vi "Otm Acquisition Loop.vi"(8 "error in (no error)":errorcluster, 9 "Data Queue":refnum<queue>, 10 "Data Notifier":refnum<notifier>, 11 "Message Queues":T1) -> (0 "error out":errorcluster)   [LabVIEW 2017]
doc: "Message loop for handling messages pertaining to the acquisition of data from the hardware."
uses:
  support/Message Queue/All Message Queues.ctl
  support/Message Queue/Message Cluster.ctl
  Acquisition/Hardware Configuration.ctl
  Acquisition/Signal Type.ctl
  Acquisition/Acquisition State.ctl
  support/Message Queue/Enqueue Message (Single).vi
  <vilib>/Utility/error.llb/Error Cluster From Error Code.vi
  <vilib>/ErrorRing/Error Ring.xnode
  Acquisition/Acquisition.lvlib
  support/Message Queue/Message Queue.lvlib
panel:
  in  "扫描频率":dbl
  out "运行时间":dbl
  in  "测试时间":dbl=30.0
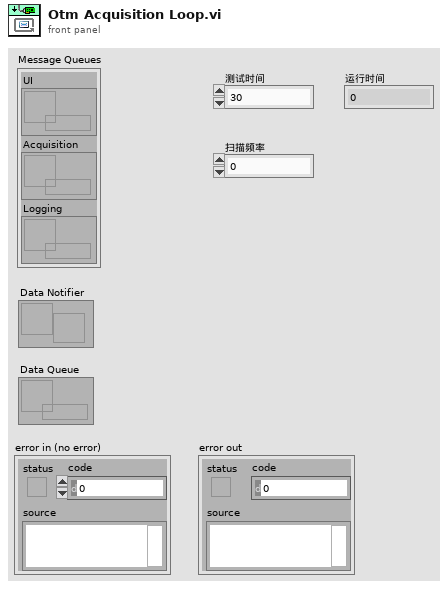
[diagram p1: front panel]
types:
  T1 = typedef "Message Queue.lvlib/All Message Queues.ctl" = cluster{"UI":refnum<queue>, "Acquisition":refnum<queue>, "Logging":refnum<queue>}
  T2 = typedef "Acquisition.lvlib/Hardware Configuration.ctl" = cluster{"HW Refnum <Replace Me>":string, "Signal Type <Replace Me>":T3}
  T3 = typedef "Acquisition.lvlib/Signal Type.ctl" = enum16{"Sine Wave", "Square with Noise"}
  T4 = typedef "Acquisition.lvlib/Acquisition State.ctl" = enum16{"Idle", "Acquiring"}
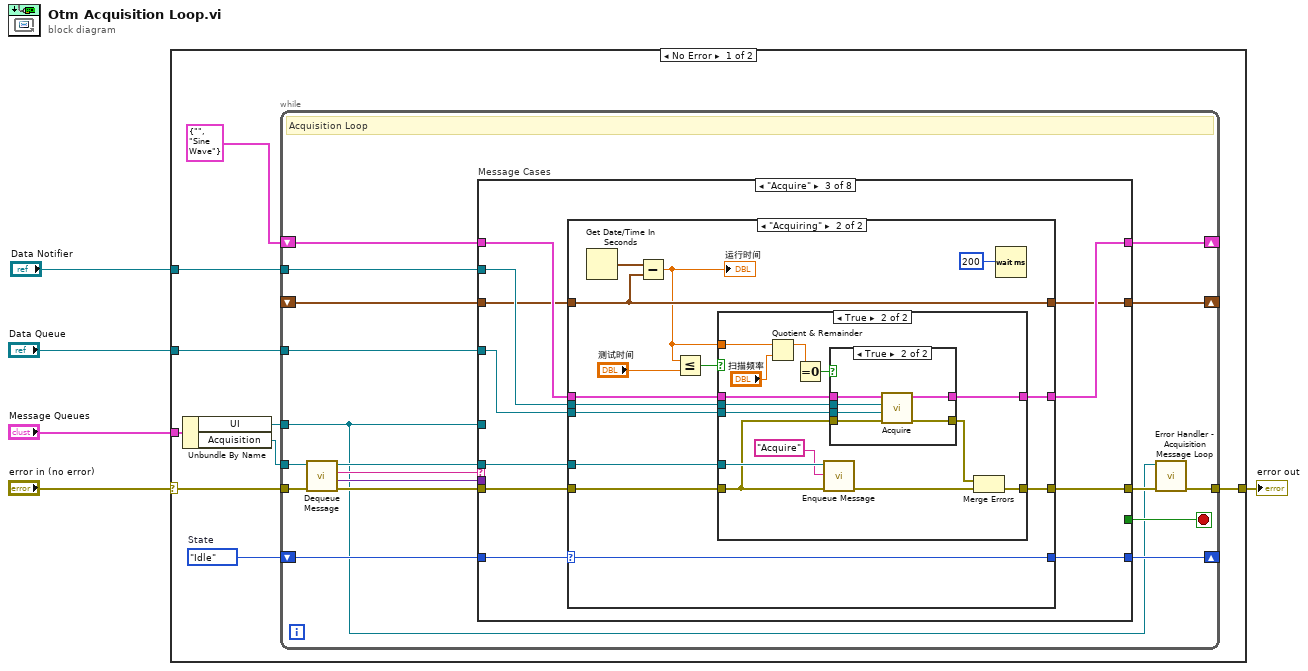
[diagram p0: block diagram]
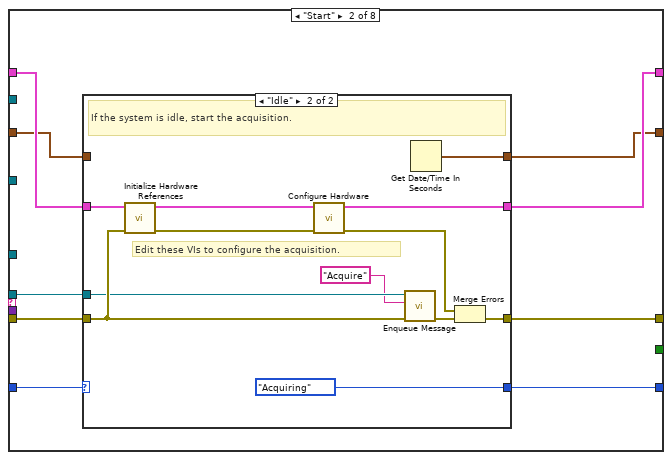
[diagram p3: hidden frame]
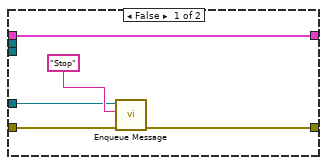
[diagram p6: hidden frame]
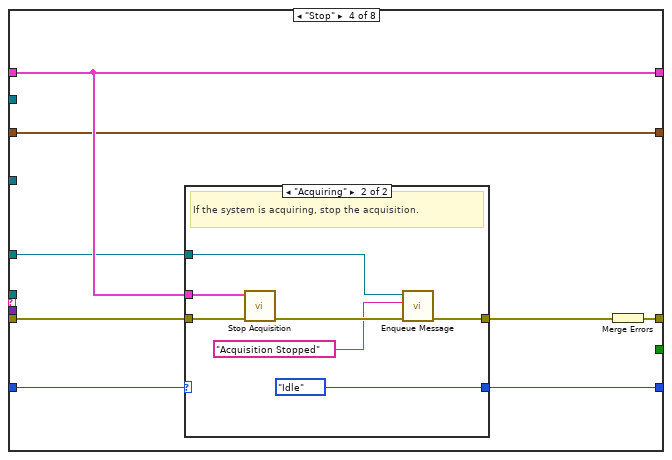
[diagram p8: hidden frame]
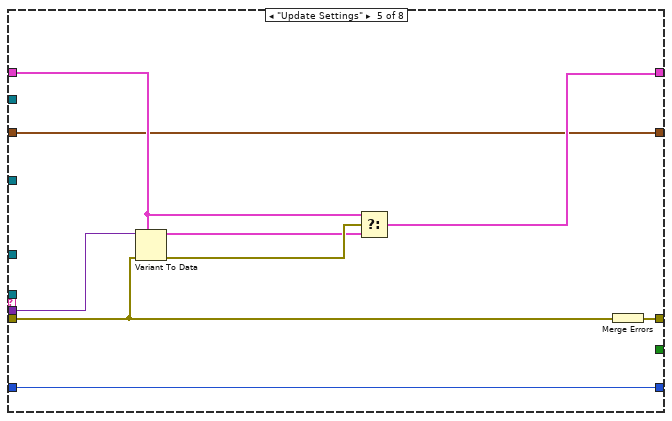
[diagram p10: hidden frame]
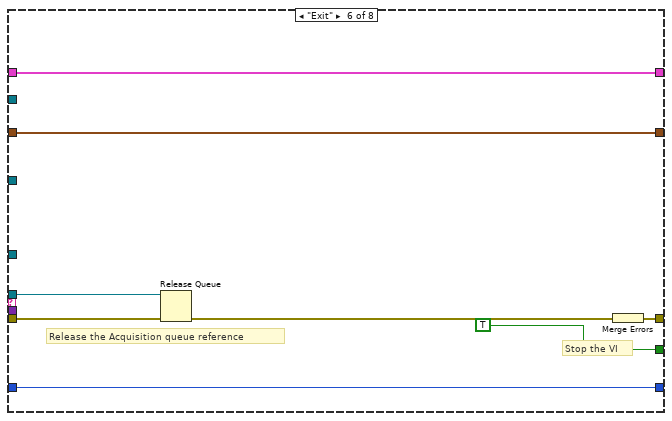
[diagram p11: hidden frame]
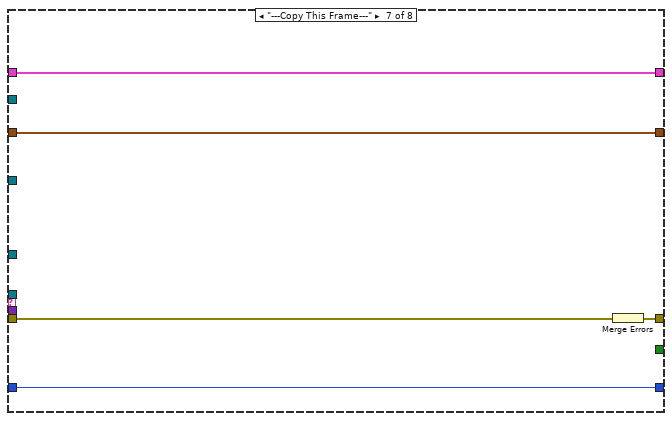
[diagram p12: hidden frame]
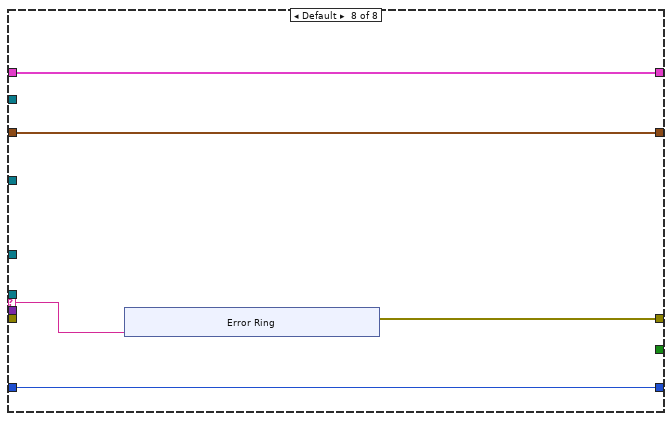
[diagram p13: hidden frame]
diagram:
  n1 = case shown="No Error" "error in (no error)" {
    selector: "error in (no error)" -> [w10 w169]
    tunnel: "Message Queues" -> [w14 _]
    tunnel: [w12 w169] -> w4
    tunnel: "Data Notifier" -> [w8 _]
    tunnel: "Data Queue" -> [w7 _]
    frame No Error {
      w6 = Acquisition_State."Idle"  # State
      n2 = Unbundle By Name(w14) -> ("UI"=w9:refnum<queue>, "Acquisition"=w13:refnum<queue>)
      n3 = while {
        tunnel: w13 -> [w25]
        shift-right: [w31] -> _
        shift-left: T2 {"HW Refnum <Replace Me>"="", "Signal Type <Replace Me>"=enum."Sine Wave"} ("Data Cluster") -> [w32]
        tunnel: w9 -> [w17]
        tunnel: w8 -> [w24]
        tunnel: w7 -> [w23]
        shift-right: [w21] -> _
        shift-left: w6 -> [w22]
        tunnel: w10 -> [w29]
        tunnel: [w20] -> w12
        shift-right: [w16] -> _
        shift-left: _ -> [w15]
        stop <- w30 stop-if-true
        # "Acquisition Loop"
        n4 = call "Dequeue Message.vi"("error in (no error)"=w29, "Message Queue"=w25) -> ("error out"=w28:errorcluster, "Message Data"=w26:variant, "Message"=w27:string, "dup Message Queue"=w18:refnum<queue>)  [unwired: 6 in]
        n5 = case "Message Cases" shown="\"Acquire\"" w27 {
          selector: w27 -> [_ _ _ _ _ _ _ w158]
          tunnel: w18 -> [_ w42 w71 _ _ w146 _ _]
          tunnel: w28 -> [w36 w43 w70 w124 w137 w148 w156 _]
          tunnel: [w36 w45 w72 w125 w143 w150 w154 w159] -> w19
          tunnel: w32 -> [w35 w44 w68 w122 w139 w149 w155 w161]
          tunnel: [w35 w41 w69 w122 w138 w149 w155 w161] -> w31
          tunnel: [_ _ _ _ _ TRUE _ _] -> w30
          tunnel: w26 -> [_ _ _ _ w142 _ _ _]
          tunnel: w17 -> [_ _ _ w119 _ _ _ _]
          tunnel: w24 -> [_ _ w67 _ _ _ _ _]
          tunnel: w23 -> [_ _ w66 _ _ _ _ _]
          tunnel: w22 -> [w34 w39 w64 w121 w136 w145 w153 w160]
          tunnel: [w34 w40 w65 w120 w136 w145 w153 w160] -> w21
          tunnel: [w33 w38 w62 w118 w135 w144 w152 w157] -> w16
          tunnel: w15 -> [w33 w37 w63 w118 w135 w144 w152 w157]
          frame "Initialize" {
            # "Initialize  - Initialize is currently a no-op.  The hardware initialization takes place in the 'Start' message."
          }
          frame "Start" {
            # "Start - Configure and start the acquisition."
            n6 = case shown="\"Idle\"" w39 {
              selector: w39 -> [w47 _]
              tunnel: [w48 w61] -> w45
              tunnel: w44 -> [w49 w60]
              tunnel: w43 -> [w48 w59]
              tunnel: w42 -> [_ w57]
              tunnel: [w49 w53] -> w41
              tunnel: [w47 Acquisition_State."Acquiring" ("Acquisition State")] -> w40
              tunnel: [w46 w50] -> w38
              tunnel: w37 -> [w46 _]
              frame "Acquiring" {
                # "The system is already acquiring. Ignore the \"Start\" message."
              }
              frame "Idle" {
                # "Edit these VIs to configure the acquisition."
                # "If the system is idle, start the acquisition."
                n7 = call "Initialize Hardware References.vi"("error in (no error)"=w59, "Hardware Resources in"=w60) -> ("error out"=w56:errorcluster, "Hardware Resources out"=w54:T2)  [unwired: 8 in]
                n8 = call "Configure Hardware.vi"("error in (no error)"=w56, "Hardware Resources in"=w54) -> ("error out"=w55:errorcluster, "Hardware Resources out"=w53:T2)  [unwired: 8 in]
                n9 = call-poly "Enqueue Message.vi"("error in (no error)"=w59, "Message"="Acquire", "Message Queue"=w57) -> ("error out"=w58:errorcluster)  [unwired: 7 in, 1 out]
                n10 = Get Date/Time In Seconds() -> (seconds since 1Jan1904=w50:timestamp)
                n11 = Merge Errors(w55, w58) -> (w61:errorcluster)
              }
            }
          }
          frame "Acquire" {
            # "Acquire - Acquire data from the hardware. Since this is a continuous acquisition, this message will always message itself to run again."
            n12 = case shown="\"Acquiring\"" w64 {
              selector: w64 -> [w74 w84]
              tunnel: [w75 w90] -> w72
              tunnel: w71 -> [_ w89]
              tunnel: w70 -> [w75 w83]
              tunnel: [w76 w88] -> w69
              tunnel: w68 -> [w76 w87]
              tunnel: w67 -> [_ w86]
              tunnel: w66 -> [_ w85]
              tunnel: [w74 w84] -> w65
              tunnel: w63 -> [w73 w79]
              tunnel: [w73 w79] -> w62
              frame "Idle" {
                # "Ignore \"Acquire\" messages when the acquisition is idle."
              }
              frame "Acquiring" {
                # "Acquire more data while in the \"Acquiring\" state."
                n13 = Get Date/Time In Seconds() -> (seconds since 1Jan1904=w82:timestamp)
                n14 = Subtract(x=w82, y=w79) -> (x-y=w77:dbl)
                "运行时间" <- w77
                n15 = Less Or Equal?(x=w77, y="测试时间") -> (x <= y?=w80:bool)
                n16 = case shown="True" w80 {
                  tunnel: [w93 w109] -> w90
                  tunnel: w89 -> [w91 w107]
                  tunnel: [w92 w105] -> w88
                  tunnel: w87 -> [w92 w104]
                  tunnel: w86 -> [_ w102]
                  tunnel: w85 -> [_ w101]
                  tunnel: w83 -> [w94 w100]
                  tunnel: w77 -> [_ w99]
                  frame False {
                    n17 = call-poly "Enqueue Message.vi"("error in (no error)"=w94, "Message"="Stop", "Message Queue"=w91) -> ("error out"=w93:errorcluster)  [unwired: 7 in, 1 out]
                  }
                  frame True {
                    n18 = Quotient & Remainder(x=w99, y="扫描频率") -> (x-y*floor(x/y)=w97:dbl)  [unwired: 1 out]
                    n19 = Equal To 0?(x=w97) -> (x = 0?=w96:bool)
                    n20 = call-poly "Enqueue Message.vi"("error in (no error)"=w100, "Message"="Acquire", "Message Queue"=w107) -> ("error out"=w108:errorcluster)  [unwired: 7 in, 1 out]
                    n21 = case shown="True" w96 {
                      tunnel: [w110 w117] -> w106
                      tunnel: [w111 w116] -> w105
                      tunnel: w104 -> [w111 w115]
                      tunnel: w102 -> [_ w114]
                      tunnel: w101 -> [_ w113]
                      tunnel: w100 -> [w110 w112]
                      frame False {
                      }
                      frame True {
                        n22 = call "Acquire.vi"("error in (no error)"=w112, "Data Queue"=w113, "Data Notifier"=w114, "Hardware Resources in"=w115) -> ("error out"=w117:errorcluster, "Hardware Resources out"=w116:T2)  [unwired: 6 in]
                      }
                    }
                    n23 = Merge Errors(w106, w108) -> (w109:errorcluster)
                  }
                }
                n24 = Wait (ms)(milliseconds to wait=u32 200) -> ()  [unwired: 1 out]
              }
            }
          }
          frame "Stop" {
            # "Stop - Stop the Acquisition."
            n25 = case shown="\"Acquiring\"" w121 {
              selector: w121 -> [w126 _]
              tunnel: w124 -> [w127 w134]
              tunnel: [w127 w130] -> w123
              tunnel: w122 -> [_ w132]
              tunnel: [w126 Acquisition_State."Idle" ("State")] -> w120
              tunnel: w119 -> [_ w129]
              frame "Idle" {
                # "The system is already idle. Ignore the \"Stop\" message."
              }
              frame "Acquiring" {
                # "If the system is acquiring, stop the acquisition."
                n26 = call "Stop Acquisition.vi"("error in (no error)"=w134, "Hardware Resources in"=w132) -> ("error out"=w133:errorcluster)  [unwired: 9 in]
                n27 = call-poly "Enqueue Message.vi"("error in (no error)"=w133, "Message"="Acquisition Stopped", "Message Queue"=w129) -> ("error out"=w130:errorcluster)  [unwired: 7 in, 1 out]
              }
            }
            n28 = Merge Errors(w123) -> (w125:errorcluster)
          }
          frame "Update Settings" {
            # "New settings are available, update the current ones stored in the shift register with the settings sent as part of the message"
            n29 = Variant To Data(error in=w137, type=w139, Variant=w142) -> (data=w140:T2, error out=w141:errorcluster)
            n30 = Select(t=w139, s=w141, f=w140) -> (s? t:f=w138:T2)
            n31 = Merge Errors(w137) -> (w143:errorcluster)
          }
          frame "Exit" {
            # "Release the Acquisition queue reference"
            # "Stop the VI"
            # "Exit - Send the Exit message to the UI Message Handler."
            n32 = Release Queue(queue=w146, error in (no error)=w148) -> (error out=w147:errorcluster)  [unwired: 1 in, 2 out]
            n33 = Merge Errors(w147) -> (w150:errorcluster)
          }
          frame "---Copy This Frame---" {
            # "Duplicate this frame when creating new messages.  Change this comment in the duplicated frame to describe this message."
            n34 = Merge Errors(w156) -> (w154:errorcluster)
          }
          frame Default {
            # "'Default' case only runs if there is a message that isn't defined in any of the other cases.  Output a programming error."
            n35 = xnode "Error Ring"("parameter 0"=w158) -> ("error out"=w159:errorcluster)
          }
        }
        n36 = call "Error Handler - Acquisition Message Loop.vi"("error in (no error)"=w19, "Message Queue"=w17) -> ("dup error in"=w20:errorcluster)  [unwired: 8 in, 1 out]
      }
    }
    frame Error {
    }
  }
  "error out" <- w4
